vi "Transmitter.vi"() -> ()   [LabVIEW 2013]
uses:
  <vilib>/addons/Modulation/Digital/General/MT Generate PSK System Parameters(M).vi
  <instrlib>/niUSRP/niUSRP Write Tx Data (CDB Cluster).vi
  <vilib>/addons/Modulation/niDMT.lvlib
panel:
  in  "Packet Parameters":T1={"Guard Bits "=30, "Sync Bits"=20, "Message Bits"=128}
  out "Number of Packets":i16=25000
  in  "Pulse Shaping Filter Parameters":T2={"Alpha"=0.5, "Filter Length"=6, "TX Filter"=enum."Root Raised Cos"} {"Alpha" format="%.2f"}
  out "Actual Tx Parameters":T3={"Tx IQ Sampling\nRate [s/sec]"=400000.0, "Tx Frequency [Hz]"=915000000.0, "Tx Gain [dB]"=20.0, "Tx Antenna"=""} {"Tx Gain [dB]" format="%#.6p"; "Tx Frequency [Hz]" format="%#.6p"; "Tx IQ Sampling\nRate [s/sec]" format="%#.6p"}
  in  "Tx Parameters":T3={"Tx IQ Sampling\nRate [s/sec]"=400000.0, "Tx Frequency [Hz]"=2330000000.0, "Tx Gain [dB]"=0.0, "Tx Antenna"="TX1"} {"Tx Gain [dB]" format="%#.6p"; "Tx Frequency [Hz]" format="%#.6p"; "Tx IQ Sampling\nRate [s/sec]" format="%#.6p"}
  in  "USRP IP Address":refnum<k15>="192.168.10.2"
  in  "Modulation Type":string(combo)="QPSK"
  out "Constellation Graph":T4(graph)
  out "Transmitted Signal":cluster{"t0":dbl, "dt":dbl, "Y":dbl[]}(graph)
  out "Error Out":errorcluster={"status"=FALSE, "code"=1074118647, "source"="niUSRP Fetch Rx Data (CDB Cluster).vi<ERR>Overflow: an internal receive buffer has filled before the data could be returned.  Consider reducing the IQ rate, increasing the Fetch rate, or increasing the number of samples per Fetch."}
  out "Symbol Rate [symbols/sec]":dbl=25000.0 format="%#.6p"
  in  "PN Sequence Order for Sync":i32=31
  in  "Stop":bool
  in  "Message Text":string="Result and Analysis：\n1、数据包的复基带波形（包格式，重点说明包头的作用）；\n2、基于队列的文本传输仿真（QPSK、整体程序框图、子VI程序框图、结果分析、生产者-消费者模型）；\n3、基于USRP的文本传输 （QPSK、整体程序框图、子VI程序框图、结果分析、生产者-消费者模型） ； \n4、分析PSK调制系统的优点和缺点，阐述其社会应用价值 \n5、扩展：5选1\n      （1） 实现16-PSK、8-PSK、QPSK、BPSK四种数字调制；\n      （2） 实验研究信噪比和误码率之间的关系（需要实测结果）；\n      （3） 实验研究升余弦滚降因子alpha、带宽和误码率之间的关系 （需要实测结果） ；\n      （4） 实现ASK/FSK的文本传输；\n      （5） 实现M-PSK图像传输；"
  in  "Queue Length":i32=10
  in  "Packet Pad [samples]":i32=200
  in  "Blank Frame [samples]":i32=500
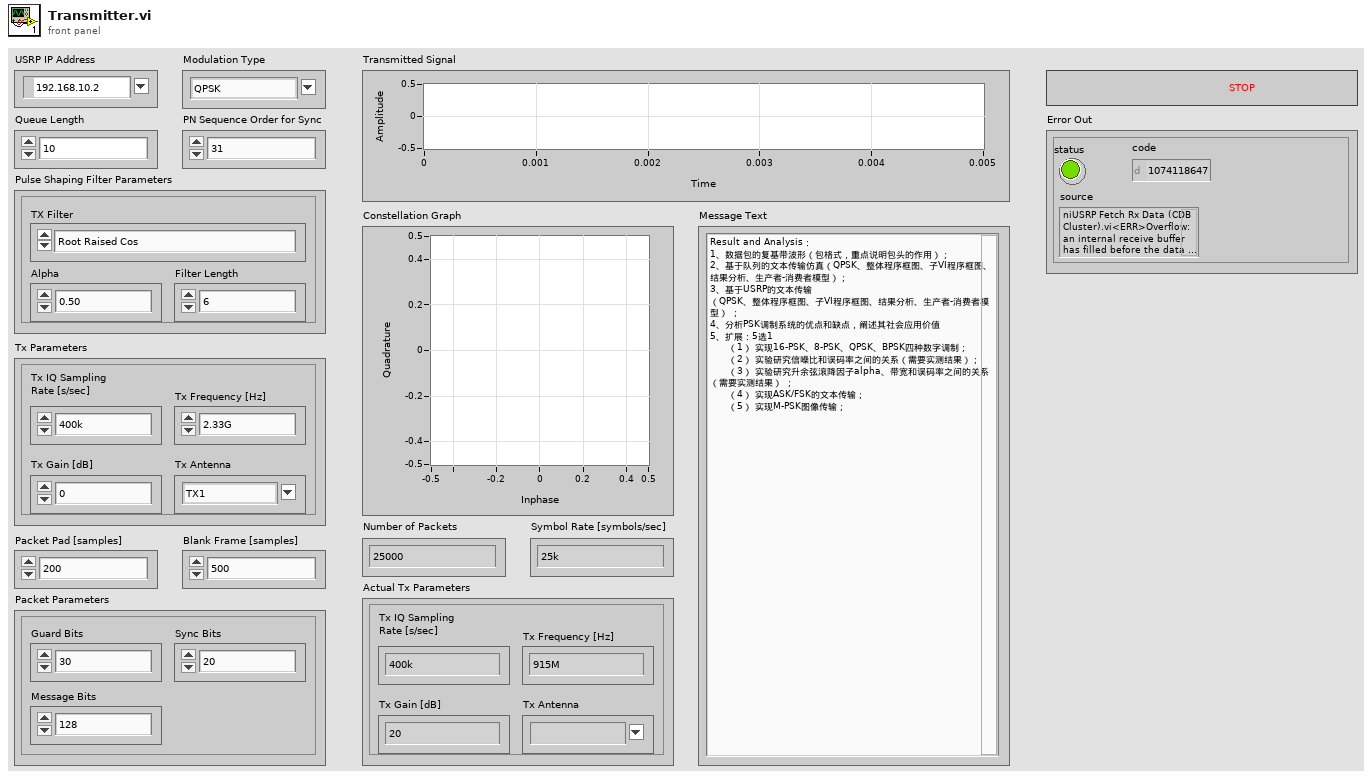
[diagram p1: front panel]
types:
  T1 = cluster{"Guard Bits ":i32, "Sync Bits":i32, "Message Bits":i32}
  T2 = cluster{"Alpha":dbl, "Filter Length":i32, "TX Filter":enum16{"none", "Raised Cosine", "Root Raised Cos", "Gaussian"}}
  T3 = cluster{"Tx IQ Sampling\nRate [s/sec]":dbl, "Tx Frequency [Hz]":dbl, "Tx Gain [dB]":dbl, "Tx Antenna":string}
  T4 = cluster{"constellation":dbl[], "oversampled data":dbl[]}[]
  T5 = cluster{"PSK type":u16, "Samples per Symbol":i32, "Differential PSK":enum16{"disable", "enable"}, "M":i32}
  T6 = cluster{"samples per symbol (16)":i32, "symbol map":cdb[], "differential PSK":enum16{"disable", "enable"}, "PSK type":u16}
  T7 = cluster{"s? t:f":cluster{"t0":dbl, "dt":dbl, "Y":cdb[]}, i32}
  T8 = cluster{"output complex waveform":cluster{"t0":dbl, "dt":dbl, "Y":cdb[]}, i32}
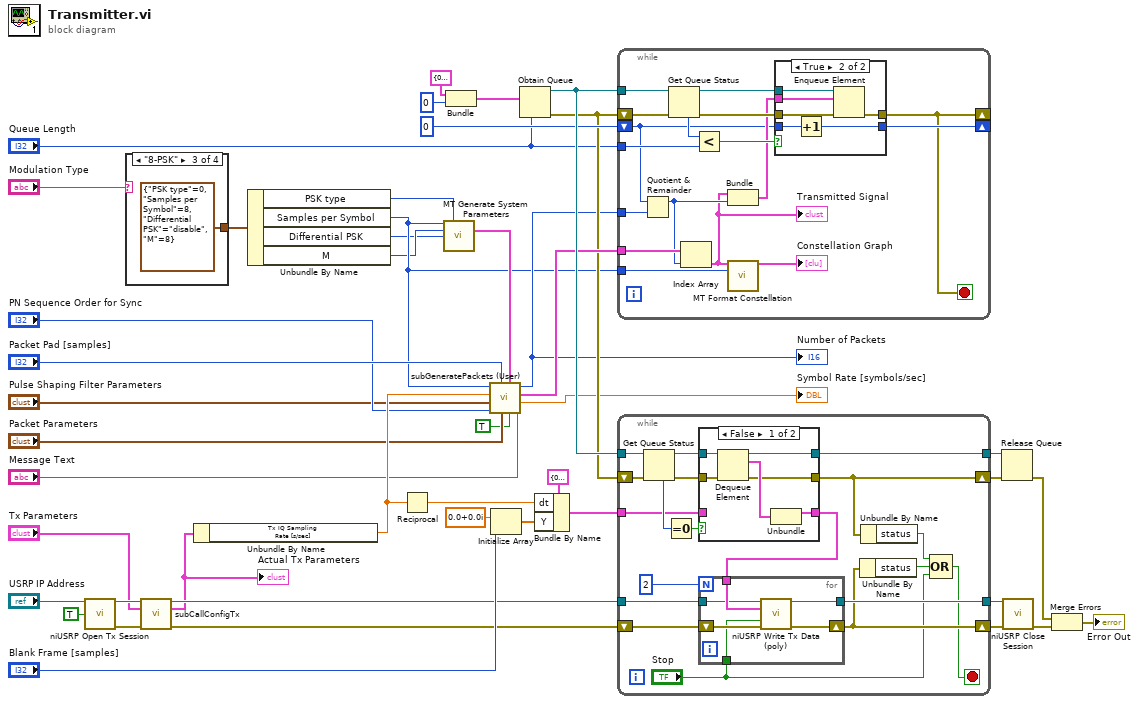
[diagram p0: block diagram]
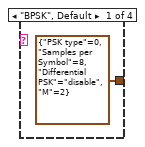
[diagram p2: hidden frame]
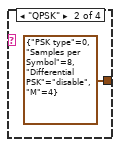
[diagram p3: hidden frame]
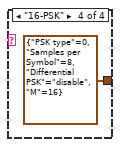
[diagram p4: hidden frame]
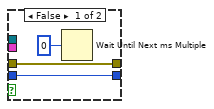
[diagram p5: hidden frame]
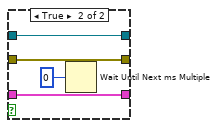
[diagram p6: hidden frame]
diagram:
  n1 = call <instrlib>:"niUSRP Open Tx Session.vi"("device names"="USRP IP Address", "reset"=TRUE) -> ("session handle out"=w26:refnum<k15>, "error out"=w25:errorcluster)  [unwired: 12 in]
  n2 = case shown="\"8-PSK\"" "Modulation Type" {
    tunnel: [T5 {"PSK type"=0, "Samples per Symbol"=8, "Differential PSK"=enum."disable", "M"=2} ("PSK Parameters") T5 {"PSK type"=0, "Samples per Symbol"=8, "Differential PSK"=enum."disable", "M"=4} ("PSK Parameters") T5 {"PSK type"=0, "Samples per Symbol"=8, "Differential PSK"=enum."disable", "M"=8} ("PSK Parameters") T5 {"PSK type"=0, "Samples per Symbol"=8, "Differential PSK"=enum."disable", "M"=16} ("PSK Parameters")] -> w9
    frame "BPSK", Default {
    }
    frame "QPSK" {
    }
    frame "8-PSK" {
    }
    frame "16-PSK" {
    }
  }
  n3 = call "subCallConfigTx.vi"("session handle"=w26, "Tx Parameters"="Tx Parameters", "error in"=w25) -> ("session handle out"=w30:refnum<k15>, "Actual Tx Parameters"=w18:T3, "error out"=w34:errorcluster)  [unwired: 10 in]
  "Actual Tx Parameters" <- w18
  n4 = Unbundle By Name(w18) -> ("Tx IQ Sampling\nRate [s/sec]"=w20:dbl)
  n5 = Unbundle By Name(w9) -> ("PSK type"=w8:u16, "Samples per Symbol"=w7:i32, "Differential PSK"=w5:enum16{"disable", "enable"}, "M"=w6:i32)
  n6 = Reciprocal(x=w20) -> (1/x=w31:dbl)
  n7 = call-poly <vilib>:"MT Generate System Parameters.vi"("samples per symbol (16)"=w7, "PSK type"=w8, "M-PSK (4)"=w6, "differential PSK"=w5) -> ("PSK system parameters"=w24:T6)  [unwired: 9 in, 2 out]
  n8 = Bundle("s? t:f"=cluster{"t0":dbl, "dt":dbl, "Y":cdb[]} {"t0"=0.0, "dt"=0.0, "Y"=[]}, 0) -> (w37:T7)  [unwired: 1 in]
  n9 = call "subGeneratePackets (User).vi"("Message Text"="Message Text", "Message Type"=TRUE, "PSK system parameters"=w24, "Packet Parameters"="Packet Parameters", "Packet Pad \n[samples]"="Packet Pad [samples]", "PN sequence order\nfor Sync Bits"="PN Sequence Order for Sync", "Pulse Shaping Filter Parameters"="Pulse Shaping Filter Parameters", "Tx IQ Sampling\nRate [s/sec]"=w20, "Samples per Symbol"=w7) -> ("Symbol Rate"=→"Symbol Rate [symbols/sec]":dbl, "Packets"=w35:cluster{"t0":dbl, "dt":dbl, "Y":cdb[]}[], "Number of Packets"=w14:i32)
  "Number of Packets" <- w14
  n10 = Initialize Array(cdb 0.0+0.0i ("element"), "Blank Frame [samples]") -> (w42:cdb[])
  n11 = Obtain Queue(max queue size (-1, unlimited)="Queue Length", element data type=w37) -> (queue out=w43:refnum<queue>, error out=w28:errorcluster)  [unwired: 3 in, 1 out]
  n12 = Bundle By Name(cluster=cluster{"t0":dbl, "dt":dbl, "Y":cdb[]} {"t0"=0.0, "dt"=0.0, "Y"=[]} ("s? t:f"), "dt"=w31, "Y"=w42) -> (w41:cluster{"t0":dbl, "dt":dbl, "Y":cdb[]})
  n13 = while {
    tunnel: w43 -> [w66]
    shift-right: [w59] -> _
    shift-left: 0 -> [w55]
    tunnel: w35 -> [w56]
    tunnel: "Queue Length" -> [w58]
    tunnel: w14 -> [w57]
    shift-right: [w53] -> _
    shift-left: w28 -> [w61]
    tunnel: w7 -> [w52]
    stop <- w53 stop-if-true
    n14 = Quotient & Remainder(x=w55, y=w57) -> (x-y*floor(x/y)=w54:i32)  [unwired: 1 out]
    n15 = Get Queue Status(queue=w66, error in (no error)=w61) -> (queue out=w65:refnum<queue>, error out=w62:errorcluster, # elements in queue=w64:i32)  [unwired: 1 in, 5 out]
    n16 = Index Array(array=w56, index=w54) -> (element=w50:cluster{"t0":dbl, "dt":dbl, "Y":cdb[]})
    "Transmitted Signal" <- w50
    n17 = Less?(x=w64, y=w58) -> (x < y?=w63:bool)
    n18 = Bundle("output complex waveform"=w50, w54) -> (w60:T8)  [unwired: 1 in]
    n19 = call <vilib>:"MT Format Constellation.vi"("waveform"=w50, "samples per symbol"=w52) -> ("constellation graph"=→"Constellation Graph":T4)  [unwired: 3 in, 10 out]
    n20 = case shown="True" w63 {
      tunnel: w62 -> [w67 w75]
      tunnel: w65 -> [_ w74]
      tunnel: [w67 w73] -> w53
      tunnel: w60 -> [_ w72]
      tunnel: w55 -> [w69 w71]
      tunnel: [w69 w70] -> w59
      frame False {
        n21 = Wait Until Next ms Multiple(millisecond multiple=u32 0) -> ()  [unwired: 1 out]
      }
      frame True {
        n22 = Increment(x=w71) -> (x+1=w70:i32)
        n23 = Enqueue Element(queue=w74, element=w72, error in (no error)=w75) -> (error out=w73:errorcluster)  [unwired: 1 in, 2 out]
      }
    }
  }
  n24 = while {
    tunnel: w30 -> [w85]
    shift-right: [w82] -> w33
    shift-left: w34 -> [w86]
    tunnel: w43 -> [w94]
    tunnel: w41 -> [w91]
    tunnel: [w90] -> w40
    tunnel: [w84] -> w32
    shift-right: [w79] -> w39
    shift-left: w28 -> [w87]
    stop <- w81 stop-if-true
    n25 = Get Queue Status(queue=w94, error in (no error)=w87) -> (queue out=w89:refnum<queue>, error out=w88:errorcluster, # elements in queue=w93:i32)  [unwired: 1 in, 5 out]
    n26 = Equal To 0?(x=w93) -> (x = 0?=w92:bool)
    n27 = case shown="False" w92 {
      tunnel: w91 -> [_ w110]
      tunnel: [w102 w110] -> w77
      tunnel: [w106 w108] -> w90
      tunnel: [w101 w109] -> w79
      tunnel: w89 -> [w105 w108]
      tunnel: w88 -> [w104 w109]
      frame False {
        n28 = Dequeue Element(queue=w105, error in (no error)=w104) -> (queue out=w106:refnum<queue>, element=w103:T7, error out=w101:errorcluster)  [unwired: 1 in, 1 out]
        n29 = Unbundle(w103) -> ("s? t:f"=w102:cluster{"t0":dbl, "dt":dbl, "Y":cdb[]})  [unwired: 1 out]
      }
      frame True {
        n30 = Wait Until Next ms Multiple(millisecond multiple=u32 0) -> ()  [unwired: 1 out]
      }
    }
    n31 = for {
      N: 2 -> [_]
      tunnel: w77 -> [w99]
      tunnel: w85 -> [w98]
      tunnel: [w97] -> w84
      tunnel: "Stop" -> [w96]
      shift-right: [w95] -> w82
      shift-left: w86 -> [w100]
      n32 = call-poly <instrlib>:"niUSRP Write Tx Data (poly).vi"("session handle"=w98, "data"=w99, "end of data?"=w96, "error in (no error)"=w100) -> ("session handle out"=w97:refnum<k15>, "error out"=w95:errorcluster)  [unwired: 10 in]
    }
    n33 = Unbundle By Name(w82) -> ("status"=w83:bool)
    n34 = Unbundle By Name(w79) -> ("status"=w78:bool)
    n35 = Compound Arithmetic op=OR(w78, w83, "Stop") -> (w81:bool)
  }
  n36 = Release Queue(queue=w40, error in (no error)=w39) -> (error out=w1:errorcluster)  [unwired: 3 out]
  n37 = call <instrlib>:"niUSRP Close Session.vi"("session handle"=w32, "error in (no error)"=w33) -> ("error out"=w23:errorcluster)  [unwired: 13 in]
  n38 = Merge Errors(w1, w23) -> (→"Error Out":errorcluster)
